vi "NewTarget.vi"(8 "Current y":dbl, 9 "Current x":dbl, 10 "Target y":dbl, 11 "Target x":dbl) -> (3 "new target?":bool)   [LabVIEW 2016, in "controllerLibrary.lvlib"]
doc: "Outputs a boolean if the target has hcnaged, which is used to reset an FGV timer"
uses:
  controllerLibrary.lvlib
  Controls/timer control.ctl
  Controls/initial conditions control.ctl
  Controls/tf control.ctl
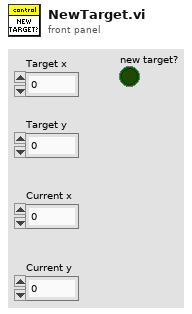
[diagram p1: front panel]
types:
  T1 = typedef "controllerLibrary.lvlib/timer control.ctl" = enum16{"get time", "set time"}
  T2 = typedef "controllerLibrary.lvlib/tf control.ctl" = enum16{"get tf", "set tf"}
  T3 = typedef "controllerLibrary.lvlib/initial conditions control.ctl" = enum16{"get", "set"}
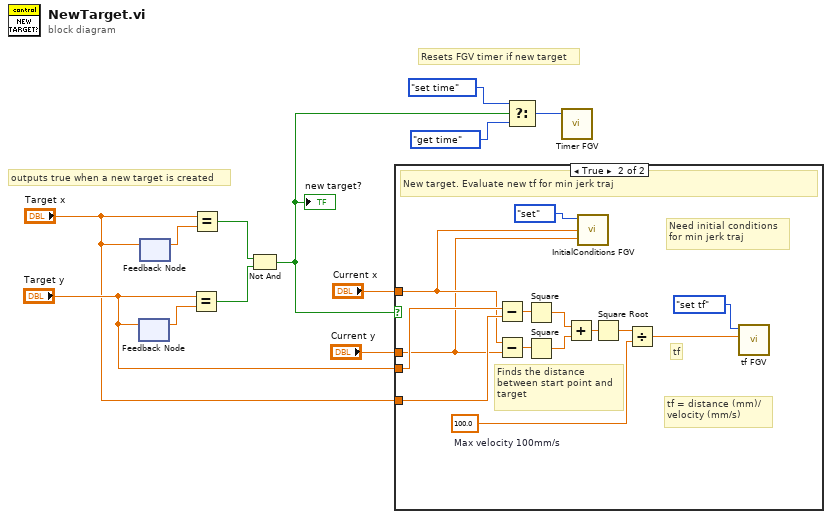
[diagram p0: block diagram]
diagram:
  # "Resets FGV timer if new target"
  # "outputs true when a new target is created"
  n1 = feedback #1() -> (w11:dbl)  [unwired: 1 in]
  n2 = feedback-in #1("Target y") -> ()
  n3 = feedback-in #2("Target x") -> ()
  n4 = feedback #2() -> (w12:dbl)  [unwired: 1 in]
  n5 = Equal?(x="Target y", y=w11) -> (x = y?=w9:bool)
  n6 = Equal?(x="Target x", y=w12) -> (x = y?=w10:bool)
  n7 = Not And(1:w9, 2:w10) -> (0:w8:bool)
  "new target?" <- w8
  n8 = case shown="True" w8 {
    tunnel: "Target y" -> [_ w21]
    tunnel: "Target x" -> [_ w20]
    tunnel: "Current y" -> [_ w15]
    tunnel: "Current x" -> [_ w16]
    frame False {
      # "Not a new target. Do nothing"
    }
    frame True {
      w18 = 100.0  # Max velocity 100mm/s
      # "Need initial conditions\nfor min jerk traj"
      # "tf = distance (mm)/\nvelocity (mm/s)"
      # "tf"
      # "Finds the distance\nbetween start point and\ntarget"
      # "New target. Evaluate new tf for min jerk traj"
      n9 = Subtract(x=w21, y=w20) -> (x-y=w26:dbl)
      n10 = Subtract(x=w16, y=w15) -> (x-y=w25:dbl)
      n11 = Square(x=w26) -> (x^2=w24:dbl)
      n12 = Square(x=w25) -> (x^2=w23:dbl)
      n13 = Add(x=w24, y=w23) -> (x+y=w22:dbl)
      n14 = call "InitialConditions FGV.vi"("Y0"=w15, "X0"=w16, "Enum"=initial_conditions_control."set") -> ()  [unwired: 7 in, 2 out]
      n15 = Square Root(x=w22) -> (sqrt(x)=w19:dbl)
      n16 = Divide(x=w19, y=w18) -> (x/y=w17:dbl)
      n17 = call "tf FGV.vi"("set tf"=w17, "Enum"=tf_control."set tf") -> ()  [unwired: 9 in, 1 out]
    }
  }
  n18 = Select(t=timer_control."set time" ("Enum"), s=w8, f=timer_control."get time" ("Enum")) -> (s? t:f=w1:T1)
  n19 = call "Timer FGV.vi"("Enum"=w1) -> ()  [unwired: 10 in, 1 out]
